vi "configure.vi"(8 "error in (no error)":errorcluster, 11 "GenericPlugin in":refnum<class "TrajectoryAK101022Resonance.lvclass">) -> (0 "error out":errorcluster, 3 "GenericPlugin out":refnum<class "TrajectoryAK101022Resonance.lvclass">)   [LabVIEW 2010, in "TrajectoryAK101022Resonance.lvclass"]
doc: "The dynamic dispatch version of this VI loads and displays the configuration file associated with the plug-in object. The user modify and save the configuration data."
uses:
  TrajectoryAK101022Resonance.lvclass
  common/xcontrols/XComponentSpecification/XComponentSpecification/XComponentSpecification.xctl
  FPGAWrapper/GenericFPGAWrapper/GenericFPGAWrapper/GenericFPGAWrapper.lvclass
  TrajectoryAK101022Resonance.lvclass/TrajectoryAK101022Resonance.ctl
  common/classes/GenericComponent/GenericComponent/GenericComponent.lvclass
panel:
  in  "z trajectory on FPGA?":bool
  in  "choose the beginning of z scan":bool
  in  "maximum z scanner value":dbl
  in  "ETL current offset":dbl[unit]=0.06
  in  "ETL current to Hifo-Box conversion":dbl[unit]=20480.0
  in  "FPGAWrapper spec":T1(xcontrol)
  in  "objective magnification":dbl
  in  "FOVx":dbl[unit]
  in  "FOVy":dbl[unit]
  in  "resonance frequency":dbl[unit]
  in  "maximum y scanner value":dbl
  in  "maximum x scanner value":dbl
  in  "scan segment default":dbl
  in  "fly-back offset default":dbl
  in  "fly-forward offset default":dbl
  in  "no. of y-brake lines after flyback":i32
  in  "no. of y-flyback lines":i32
  in  "no. of y-brake lines before flyback":i32
  in  "cancelButton":bool
  in  "saveButton":bool
  out "configuration name":string
  # "Configure TrajectoryAK101022Resonance"
  # "FPGA wrapper"
  # "Note\nMeasure the Field Of View at zoom 1x and use the stage to measure left-to-right and top-to bottom.\nIndicate at which objective magnification this is measured."
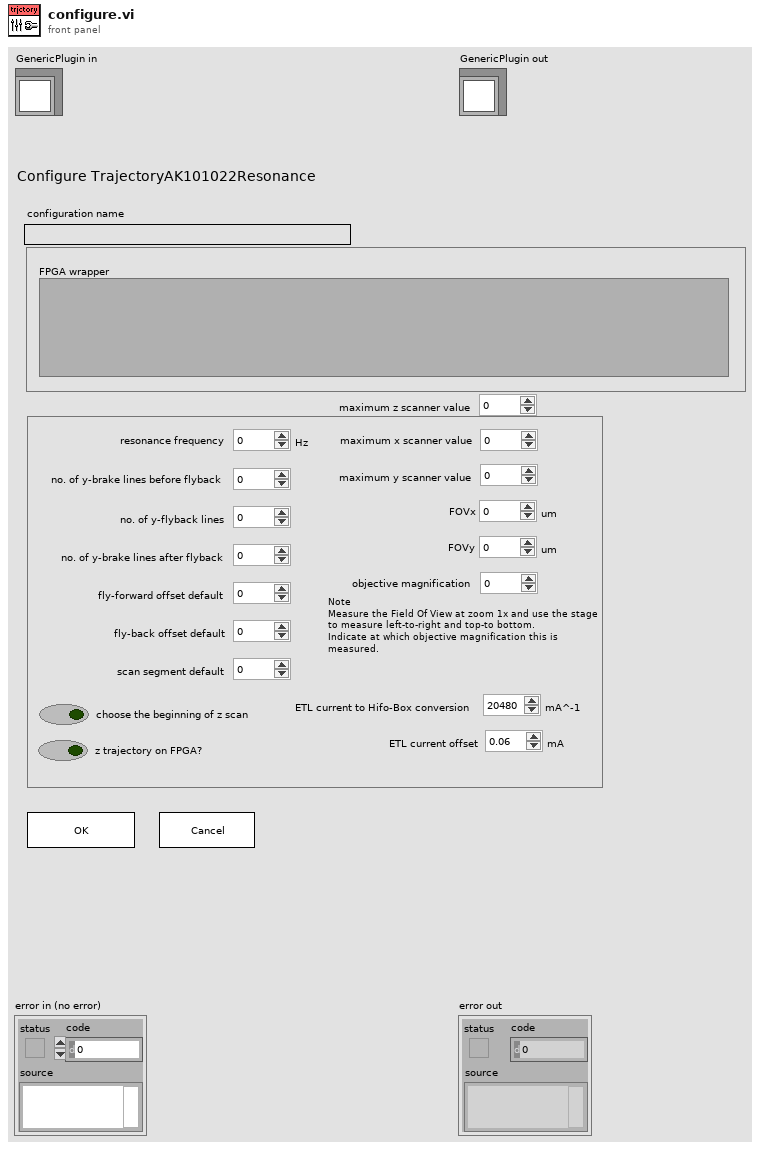
[diagram p1: front panel]
types:
  T1 = cluster{"class path":string, "configuration":string, "label":string, "settings name":string}
  T2 = typedef "plugin_specification.ctl" = cluster{"class path":string, "configuration":string, "label":string, "settings name":string}
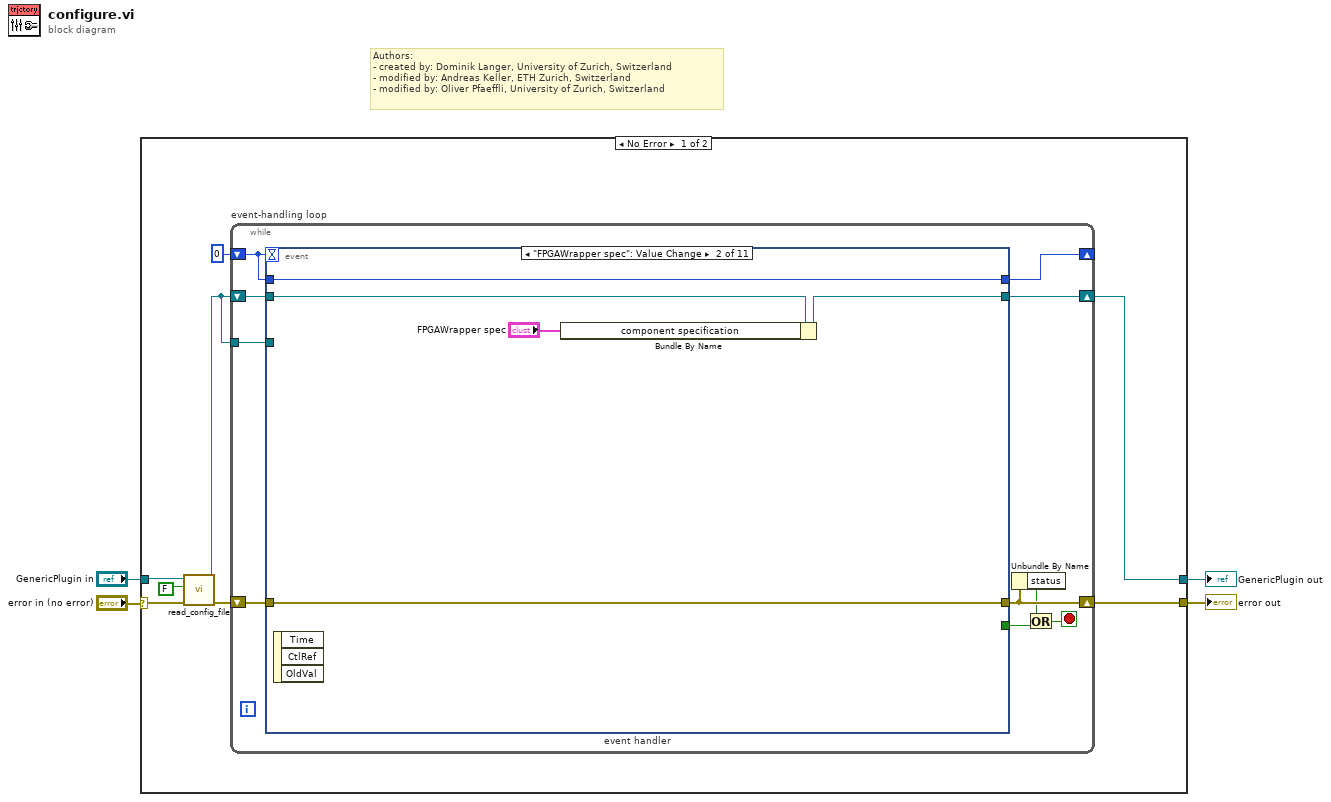
[diagram p0: block diagram]
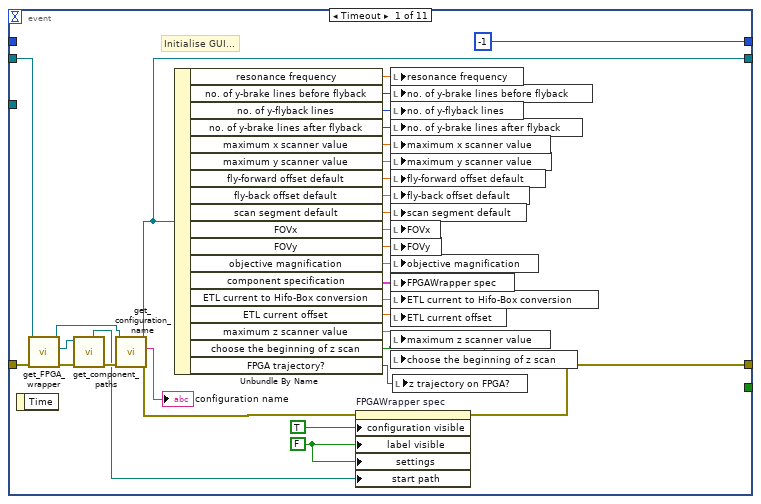
[diagram p2: hidden frame]
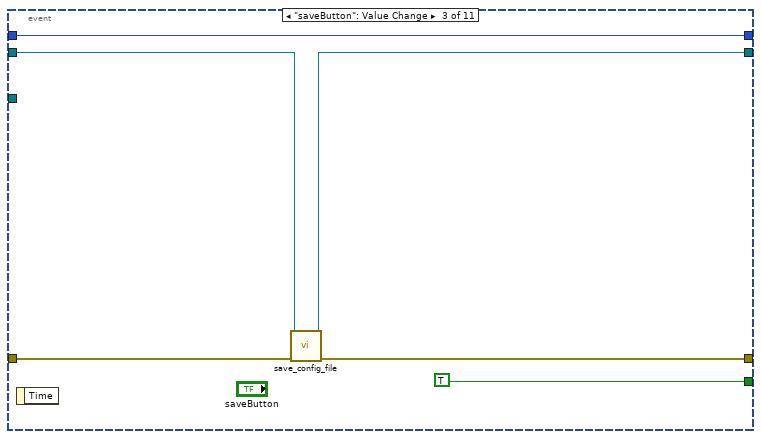
[diagram p3: hidden frame]
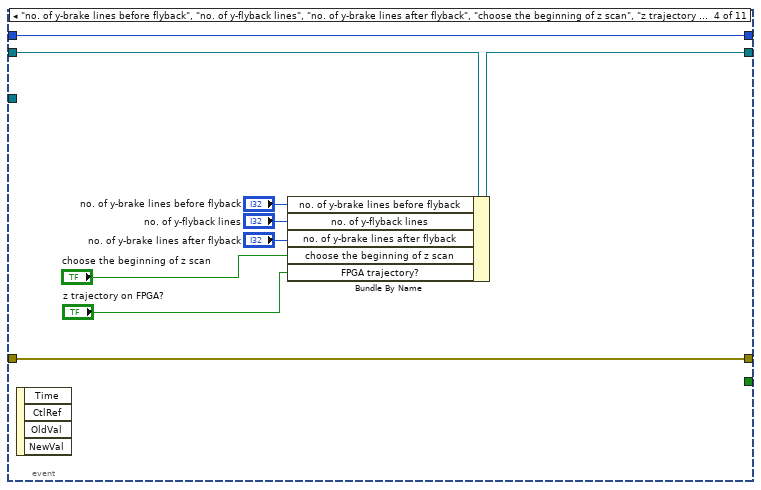
[diagram p4: hidden frame]
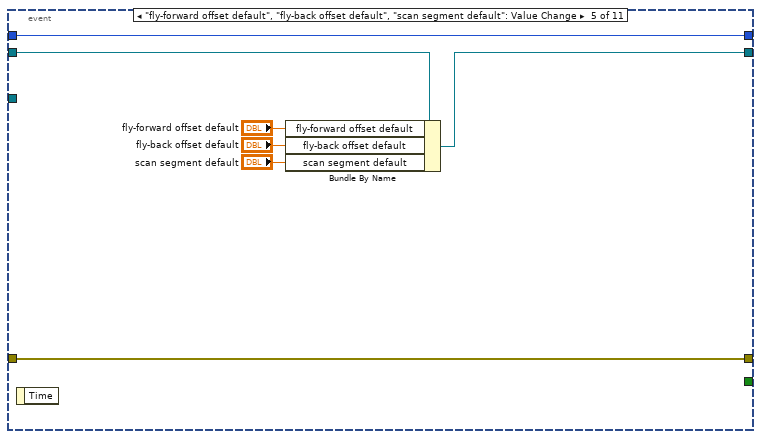
[diagram p5: hidden frame]
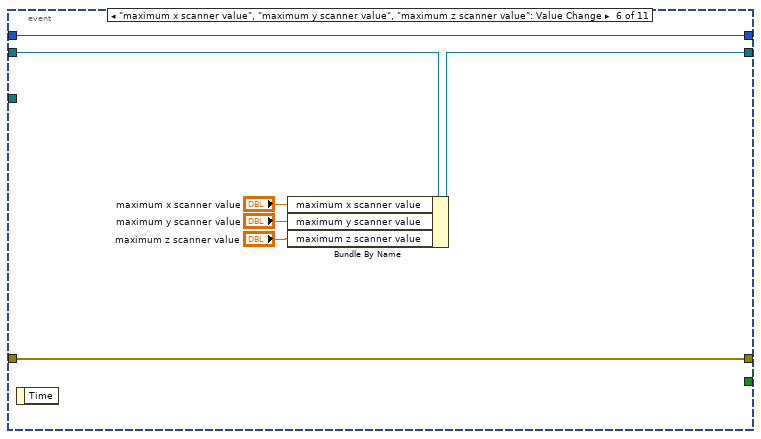
[diagram p6: hidden frame]
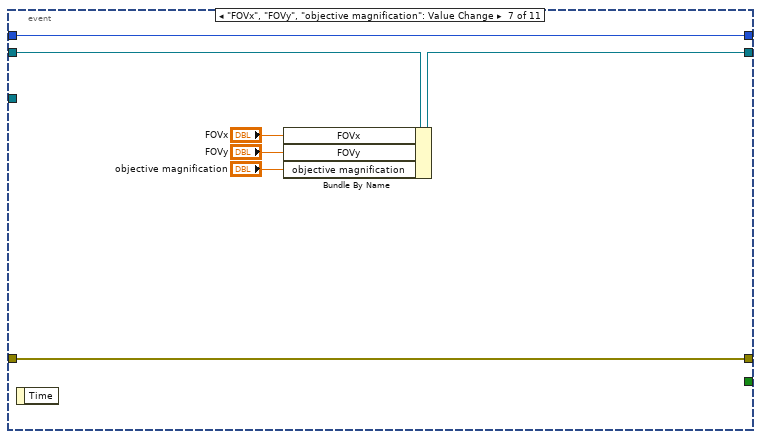
[diagram p7: hidden frame]
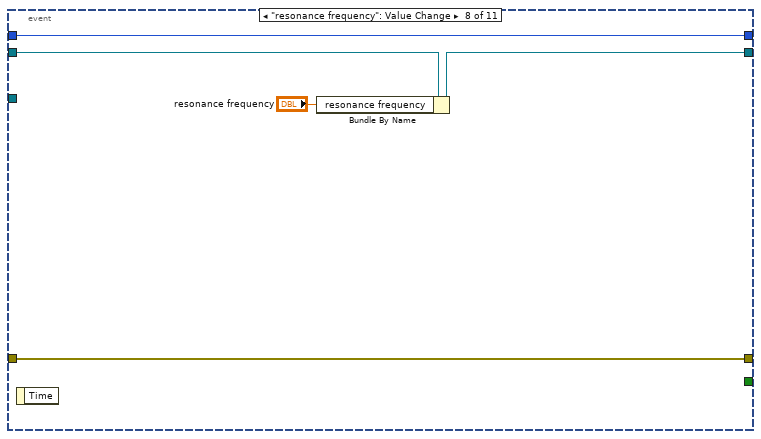
[diagram p8: hidden frame]
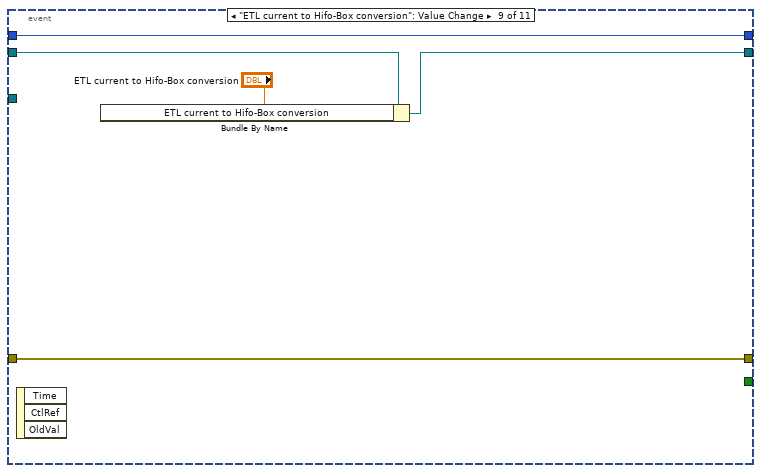
[diagram p9: hidden frame]
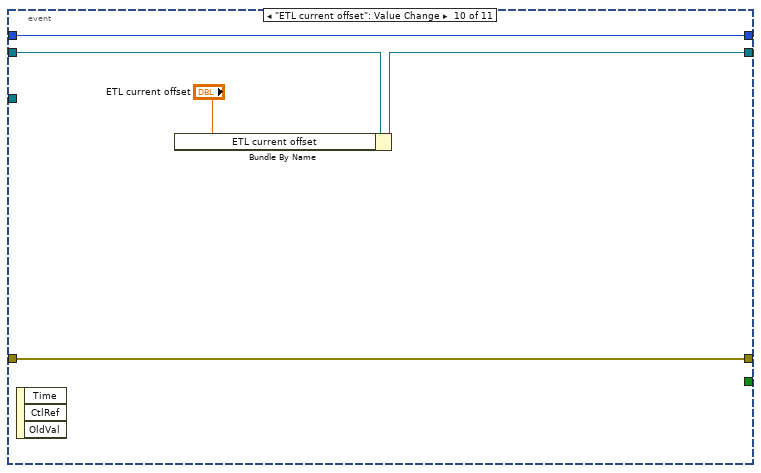
[diagram p10: hidden frame]
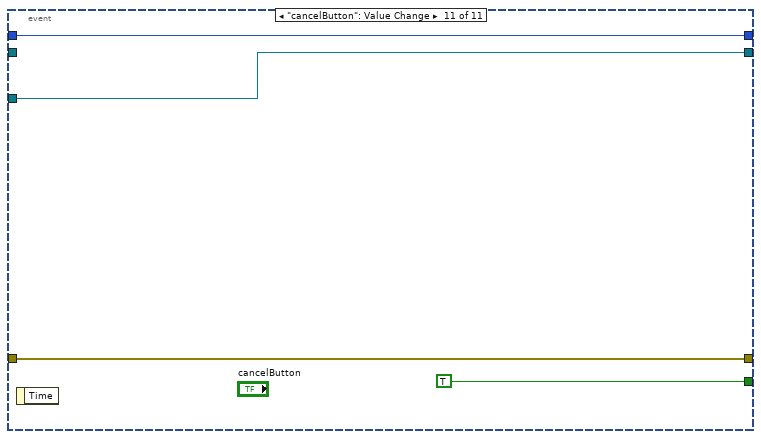
[diagram p11: hidden frame]
diagram:
  # "Authors: \n- created by: Dominik Langer, University of Zurich, Switzerland\n- modified by: Andreas Keller, ETH Zurich, Switzerland\n- modified by: Oliver Pfaeffli, University of Zurich, Switzerland"
  n1 = case shown="No Error" "error in (no error)" {
    selector: "error in (no error)" -> [w7 w115]
    tunnel: [w6 w115] -> w3
    tunnel: [w5 w116] -> w1
    tunnel: "GenericPlugin in" -> [w8 w116]
    frame No Error {
      n2 = call-dynamic "read_config_file.vi"("error in (no error)"=w7, "force load?"=FALSE, "GenericPlugin in"=w8) -> ("error out"=w12:errorcluster, "GenericPlugin out"=w11:refnum<class "TrajectoryAK101022Resonance.lvclass">)  [unwired: 7 in]
      n3 = while "event-handling loop" {
        shift-right: [w19] -> w6
        shift-left: w12 -> [w22]
        shift-right: [w20] -> w5
        shift-left: w11 -> [w21]
        tunnel: w11 -> [w15]
        shift-right: [w13] -> _
        shift-left: 0 -> [w14]
        stop <- w16 stop-if-true
        n4 = event "event handler" shown="[1] \"FPGAWrapper spec\": Value Change" {
          selector: _ -> [_ _ _ _ _ _ _ _ _ _ _]
          dyn-events: _ -> [_ _ _ _ _ _ _ _ _ _ _]
          timeout: w14 -> [_ _ _ _ _ _ _ _ _ _ _]
          tunnel: w22 -> [w36 w59 w64 w74 w81 w88 w95 w100 w105 w110 w114]
          tunnel: [w31 w59 w63 w74 w81 w88 w95 w100 w105 w110 w114] -> w19
          tunnel: w21 -> [w35 w56 w62 w73 w79 w87 w93 w99 w103 w108 _]
          tunnel: [w53 w55 w61 w72 w78 w86 w92 w98 w102 w107 w112] -> w20
          tunnel: [_ _ TRUE _ _ _ _ _ _ _ TRUE] -> w18
          tunnel: w15 -> [_ _ _ _ _ _ _ _ _ _ w112]
          tunnel: [-1 w58 w60 w71 w80 w85 w94 w97 w104 w109 w111] -> w13
          tunnel: w14 -> [_ w58 w60 w71 w80 w85 w94 w97 w104 w109 w111]
          event Timeout {
            w38 = FALSE ("label visible")
            # "Initialise GUI..."
            n5 = event-data() -> ()  [unwired: 1 in, 1 out]
            n6 = call-dynamic "get_FPGA_wrapper.vi"("error in (no error)"=w36, "TrajectoryMG100122GenericFPGA in"=w35) -> ("error out"=w34:errorcluster, "GenericFPGAWrapper.lvclass"=w29:refnum<class "GenericFPGAWrapper.lvclass">, "TrajectoryMG100122GenericFPGA out"=w28:refnum<class "TrajectoryAK101022Resonance.lvclass">)  [unwired: 7 in]
            n7 = call-dynamic "get_component_paths.vi"("error in (no error)"=w34, "GenericComponent in"=w29) -> ("error out"=w33:errorcluster, "component type directory"=w30:path)  [unwired: 4 in, 4 out]
            n8 = call "get_configuration_name.vi"("error in (no error)"=w33, "GenericPlugin.lvclass in"=w28) -> ("error out"=w32:errorcluster, "configuration name"=→"configuration name":string, "GenericPlugin.lvclass out"=w53:refnum<class "TrajectoryAK101022Resonance.lvclass">)  [unwired: 7 in]
            n9 = Unbundle By Name(w53) -> ("resonance frequency"=w51:dbl[unit], "no. of y-brake lines before flyback"=w50:i32, "no. of y-flyback lines"=w49:i32, "no. of y-brake lines after flyback"=w48:i32, "maximum x scanner value"=w47:dbl, "maximum y scanner value"=w46:dbl, "fly-forward offset default"=w45:dbl, "fly-back offset default"=w44:dbl, "scan segment default"=w43:dbl, "FOVx"=w42:dbl[unit], "FOVy"=w41:dbl[unit], "objective magnification"=w40:dbl, "component specification"=w37:T2, "ETL current to Hifo-Box conversion"=w27:dbl[unit], "ETL current offset"=w26:dbl[unit], "maximum z scanner value"=w25:dbl, "choose the beginning of z scan"=w24:bool, "FPGA trajectory?"=w23:bool)
            n10 = property on="FPGAWrapper spec" class="XComponentSpecification (strict"(error in=w32, "configuration visible"=TRUE, "label visible"=w38, "settings"=w38, "start path"=w30) -> (error out=w31:errorcluster)  [unwired: 1 in, 1 out]
            n11 = local write "resonance frequency"(w51) -> ()
            n12 = local write "no. of y-brake lines before flyback"(w50) -> ()
            n13 = local write "no. of y-flyback lines"(w49) -> ()
            n14 = local write "no. of y-brake lines after flyback"(w48) -> ()
            n15 = local write "maximum x scanner value"(w47) -> ()
            n16 = local write "maximum y scanner value"(w46) -> ()
            n17 = local write "fly-forward offset default"(w45) -> ()
            n18 = local write "fly-back offset default"(w44) -> ()
            n19 = local write "scan segment default"(w43) -> ()
            n20 = local write "FOVx"(w42) -> ()
            n21 = local write "FOVy"(w41) -> ()
            n22 = local write "objective magnification"(w40) -> ()
            n23 = local write "FPGAWrapper spec"(w37) -> ()
            n24 = local write "ETL current to Hifo-Box conversion"(w27) -> ()
            n25 = local write "ETL current offset"(w26) -> ()
            n26 = local write "maximum z scanner value"(w25) -> ()
            n27 = local write "choose the beginning of z scan"(w24) -> ()
            n28 = local write "z trajectory on FPGA?"(w23) -> ()
          }
          event "FPGAWrapper spec": Value Change {
            n29 = event-data() -> ()  [unwired: 1 in, 3 out]
            n30 = Bundle By Name(cluster=w56, "component specification"="FPGAWrapper spec") -> (w55:refnum<class "TrajectoryAK101022Resonance.lvclass">)
          }
          event "saveButton": Value Change {
            n31 = event-data() -> ()  [unwired: 1 in, 1 out]
            n32 = call-dynamic "save_config_file.vi"("error in (no error)"=w64, "GenericPlugin in"=w62) -> ("error out"=w63:errorcluster, "GenericPlugin out"=w61:refnum<class "TrajectoryAK101022Resonance.lvclass">)  [unwired: 8 in]
          }
          event "no. of y-brake lines before flyback", "no. of y-flyback lines", "no. of y-brake lines after flyback", "choose the beginning of z scan", "z trajectory on FPGA?": Value Change {
            n33 = event-data() -> ()  [unwired: 1 in, 4 out]
            n34 = Bundle By Name(cluster=w73, "no. of y-brake lines before flyback"="no. of y-brake lines before flyback", "no. of y-flyback lines"="no. of y-flyback lines", "no. of y-brake lines after flyback"="no. of y-brake lines after flyback", "choose the beginning of z scan"="choose the beginning of z scan", "FPGA trajectory?"="z trajectory on FPGA?") -> (w72:refnum<class "TrajectoryAK101022Resonance.lvclass">)
          }
          event "fly-forward offset default", "fly-back offset default", "scan segment default": Value Change {
            n35 = event-data() -> ()  [unwired: 1 in, 1 out]
            n36 = Bundle By Name(cluster=w79, "fly-forward offset default"="fly-forward offset default", "fly-back offset default"="fly-back offset default", "scan segment default"="scan segment default") -> (w78:refnum<class "TrajectoryAK101022Resonance.lvclass">)
          }
          event "maximum x scanner value", "maximum y scanner value", "maximum z scanner value": Value Change {
            n37 = event-data() -> ()  [unwired: 1 in, 1 out]
            n38 = Bundle By Name(cluster=w87, "maximum x scanner value"="maximum x scanner value", "maximum y scanner value"="maximum y scanner value", "maximum z scanner value"="maximum z scanner value") -> (w86:refnum<class "TrajectoryAK101022Resonance.lvclass">)
          }
          event "FOVx", "FOVy", "objective magnification": Value Change {
            n39 = event-data() -> ()  [unwired: 1 in, 1 out]
            n40 = Bundle By Name(cluster=w93, "FOVx"="FOVx", "FOVy"="FOVy", "objective magnification"="objective magnification") -> (w92:refnum<class "TrajectoryAK101022Resonance.lvclass">)
          }
          event "resonance frequency": Value Change {
            n41 = event-data() -> ()  [unwired: 1 in, 1 out]
            n42 = Bundle By Name(cluster=w99, "resonance frequency"="resonance frequency") -> (w98:refnum<class "TrajectoryAK101022Resonance.lvclass">)
          }
          event "ETL current to Hifo-Box conversion": Value Change {
            n43 = event-data() -> ()  [unwired: 1 in, 3 out]
            n44 = Bundle By Name(cluster=w103, "ETL current to Hifo-Box conversion"="ETL current to Hifo-Box conversion") -> (w102:refnum<class "TrajectoryAK101022Resonance.lvclass">)
          }
          event "ETL current offset": Value Change {
            n45 = event-data() -> ()  [unwired: 1 in, 3 out]
            n46 = Bundle By Name(cluster=w108, "ETL current offset"="ETL current offset") -> (w107:refnum<class "TrajectoryAK101022Resonance.lvclass">)
          }
          event "cancelButton": Value Change {
            n47 = event-data() -> ()  [unwired: 1 in, 1 out]
          }
        }
        n48 = Unbundle By Name(w19) -> ("status"=w17:bool)
        n49 = Or(x=w17, y=w18) -> (x .or. y?=w16:bool)
      }
    }
    frame Error {
    }
  }
  "error out" <- w3
  "GenericPlugin out" <- w1
